vi "NI PXIe-411x PS Main Page.vi"(8 "error in (no error)":errorcluster, 11 "Node Ptr":T1 format="%.0x") -> (0 "error out":errorcluster)   [LabVIEW 2023, in "NI PXIe-411x PS Custom Device.lvlib"]
uses:
  NI PXIe-411x PS Custom Device.lvlib
  <vilib>/NI VeriStand/Custom Device API/Custom Device Item Ref.ctl
  411x_Global.vi
  <vilib>/NI VeriStand/Custom Device API/Get Item Property (String).vi
  <vilib>/NI VeriStand/Custom Device API/Get Item Property (Boolean).vi
  <vilib>/NI VeriStand/Custom Device API/Set Item Property (String).vi
  <vilib>/NI VeriStand/Custom Device API/Set Item Property (Boolean).vi
  <vilib>/NI VeriStand/Custom Device API/Custom Device API.lvlib
panel:
  in  "Module":bool=TRUE
  in  "HW Device Name in MAX":string
  in  "Add Current Chans":bool
  in  "Add Voltage Chans":bool
  in  "Header":cluster{"Section Name":string}={"Section Name"="PXIe-411x  Settings"}
  in  "Description":string
  in  "Custom Device Name":string
  in  "Delete":bool
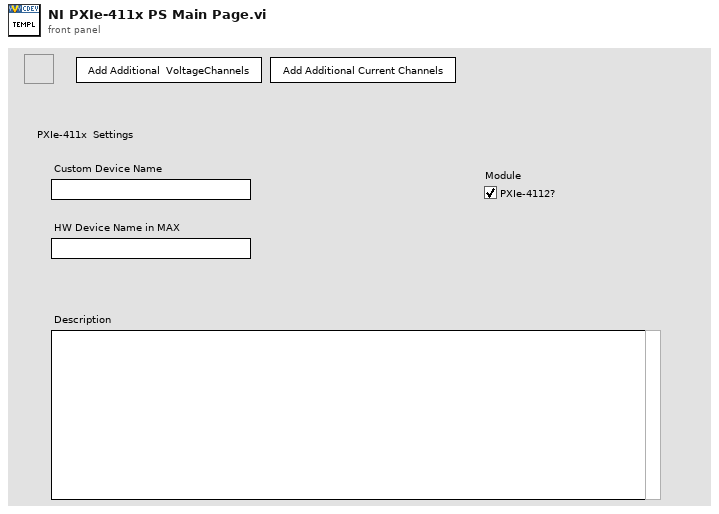
[diagram p1: front panel]
types:
  T1 = typedef "Custom Device API.lvlib/Custom Device Item Ref.ctl" = u64
  T2 = typedef "Custom Device API.lvlib/Custom Device Item Info.ctl" = cluster{"Name":string, "Is Channel":bool, "GUID":string, "Is Waveform":bool}
  T3 = typedef "Custom Device API.lvlib/Custom Device Commands.ctl" = enum16{"Default", "Item renamed", "Shutdown", "Dynamic button pressed"}
  T4 = typedef "niDCPower Sense.ctl" = i32
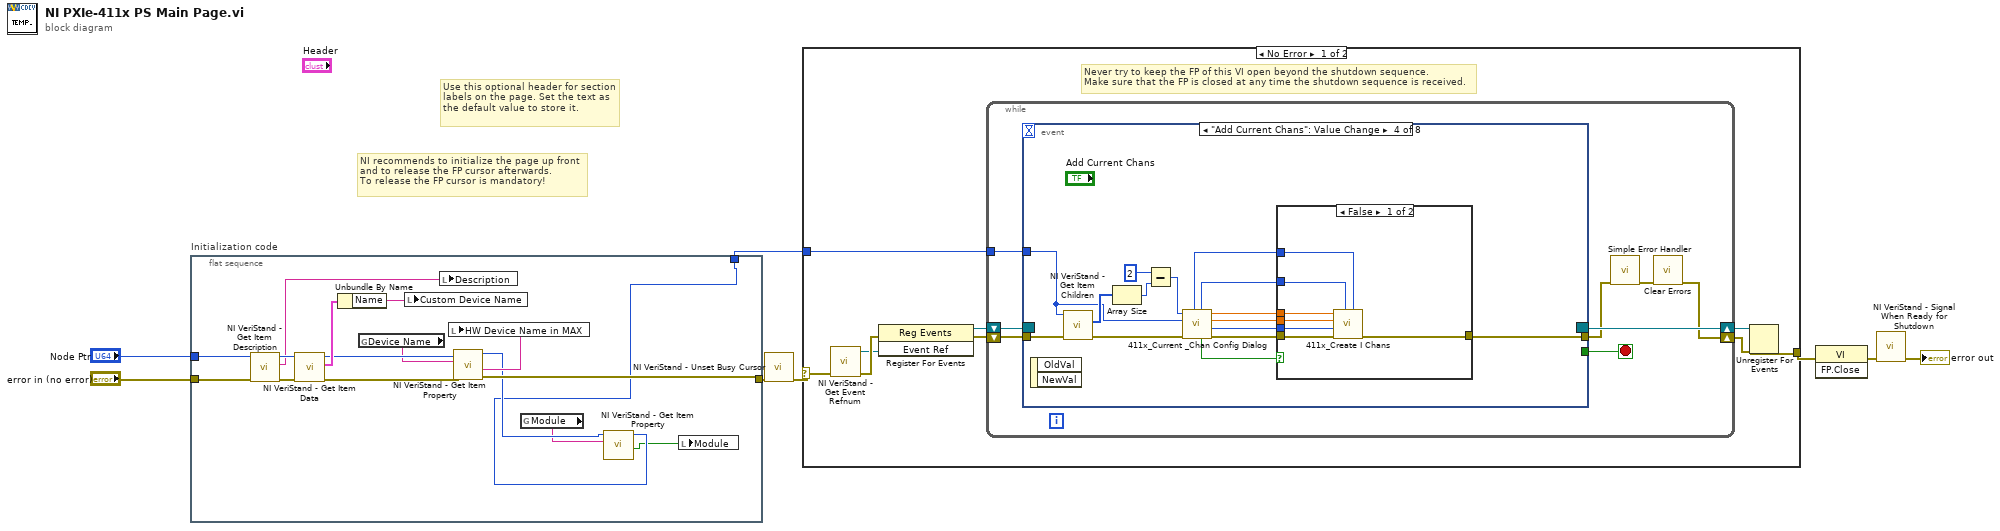
[diagram p0: block diagram]
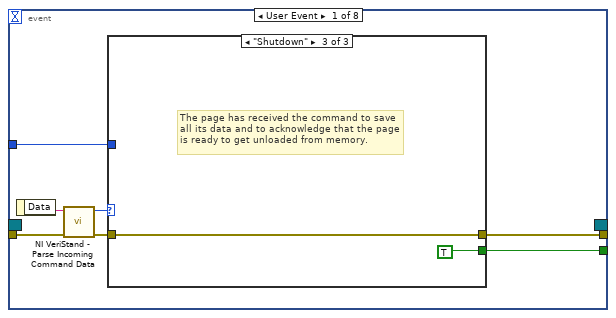
[diagram p2: hidden frame]
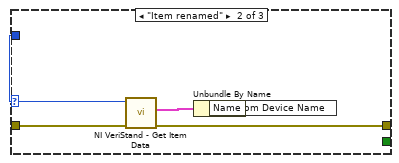
[diagram p4: hidden frame]
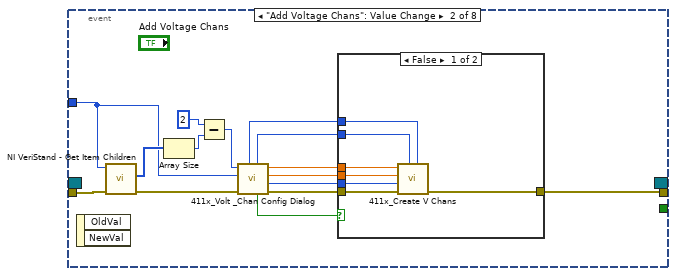
[diagram p5: hidden frame]
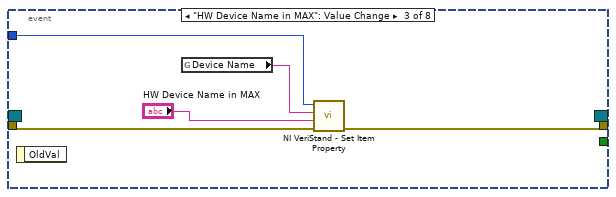
[diagram p7: hidden frame]
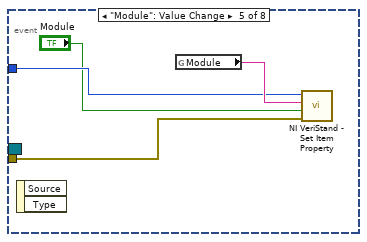
[diagram p9: hidden frame]
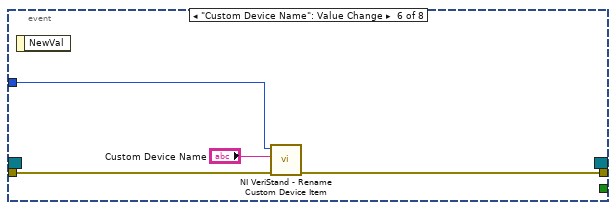
[diagram p10: hidden frame]
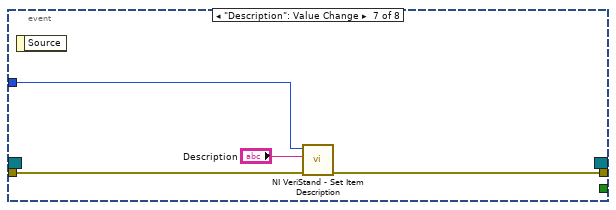
[diagram p11: hidden frame]
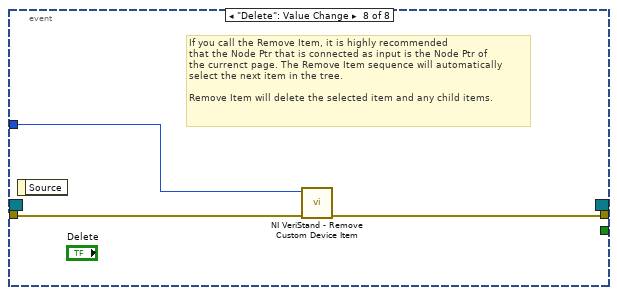
[diagram p12: hidden frame]
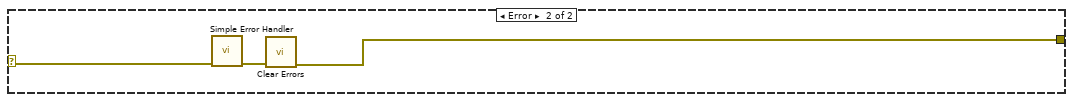
[diagram p13: hidden frame]
diagram:
  # "Use this optional header for section labels on the page. Set the text as the default value to store it."
  # "NI recommends to initialize the page up front\nand to release the FP cursor afterwards.\nTo release the FP cursor is mandatory!"
  n1 = flat-sequence "Initialization code" {
    tunnel: "error in (no error)" -> [w18]
    tunnel: "Node Ptr" -> [w19]
    tunnel: [w15] -> w4
    tunnel: [w11] -> w1
    frame #0 {
      n2 = call <vilib>:"NI VeriStand - Get Item Description.vi"("error in (no error)"=w18, "Item Ref in"=w19) -> ("error out"=w22:errorcluster, "Description"=w23:string, "Item Ref out"=w24:T1)  [unwired: 7 out]
      n3 = call <vilib>:"NI VeriStand - Get Item Data.vi"("error in (no error)"=w22, "Item Ref in"=w24) -> ("error out"=w17:errorcluster, "Item Info"=w21:T2, "Item Ref out"=w16:T1)  [unwired: 7 out]
      n4 = Unbundle By Name(w21) -> ("Name"=w20:string)
      n5 = global read "411x_Global.vi" "Device Name"() -> (w14:string)
      n6 = local write "Custom Device Name"(w20) -> ()
      n7 = local write "Description"(w23) -> ()
      n8 = call-poly <vilib>:"NI VeriStand - Get Item Property.vi"("error in (no error)"=w17, "Property Name"=w14, "Item Ref in"=w16) -> ("error out"=w15:errorcluster, "Value"=w13:string, "Item Ref out"=w12:T1)  [unwired: 5 in, 1 out]
      n9 = local write "HW Device Name in MAX"(w13) -> ()
      n10 = global read "411x_Global.vi" "Module"() -> (w10:string)
      n11 = call-poly <vilib>:"NI VeriStand - Get Item Property.vi"("Property Name"=w10, "Item Ref in"=w12) -> ("Value"=w9:bool, "Item Ref out"=w11:T1)  [unwired: 6 in, 2 out]
      n12 = local write "Module"(w9) -> ()
    }
  }
  n13 = call <vilib>:"NI VeriStand - Unset Busy Cursor.vi"("error in (no error)"=w4) -> ("error out"=w3:errorcluster)  [unwired: 10 out]
  n14 = case shown="No Error" w3 {
    selector: w3 -> [w25 w125]
    tunnel: [w30 w123] -> w8
    tunnel: w1 -> [w26 _]
    frame No Error {
      # "Never try to keep the FP of this VI open beyond the shutdown sequence.\nMake sure that the FP is closed at any time the shutdown sequence is received."
      n15 = call <vilib>:"NI VeriStand - Get Event Refnum.vi"("error in (no error)"=w25) -> ("error out"=w33:errorcluster, "Event Ref"=w29:refnum<user-event>)  [unwired: 9 out]
      n16 = register-events(error in=w33, w29) -> (reference out=w27:refnum<event-registration>, error out=w28:errorcluster)  [unwired: 1 in]
      n17 = while {
        tunnel: w26 -> [w37]
        shift-right: [w34] -> w31
        shift-left: w28 -> [w40]
        shift-right: [w41] -> w32
        shift-left: w27 -> [w39]
        stop <- w38 stop-if-true
        n18 = event shown="[3] \"Add Current Chans\": Value Change" {
          selector: w39 -> [_ _ _ _ _ _ _ _]
          dyn-events: [_ _ _ _ _ _ _ _] -> w41
          timeout: _ -> [_ _ _ _ _ _ _ _]
          tunnel: w40 -> [w48 w71 w84 w99 w108 w115 w118 w122]
          tunnel: [w44 _ _ _ _ _ _ _] -> w38
          tunnel: [w43 w60 w80 w88 _ w114 w117 w121] -> w36
          tunnel: w37 -> [w42 w58 w83 w86 w110 w113 w119 w120]
          event User Event {
            n19 = event-data() -> ("Data"=w47:string)  [unwired: 1 out]
            n20 = call <vilib>:"NI VeriStand - Parse Incoming Command Data.vi"("error in (no error)"=w48, "Incoming data"=w47) -> ("error out"=w46:errorcluster, "Action"=w45:T3)  [unwired: 8 out]
            n21 = case shown="\"Shutdown\"" w45 {
              tunnel: w46 -> [w49 w54 w55]
              tunnel: [_ _ TRUE] -> w44
              tunnel: [w49 w51 w55] -> w43
              tunnel: w42 -> [_ w53 _]
              frame "Default", Default {
              }
              frame "Item renamed" {
                n22 = call <vilib>:"NI VeriStand - Get Item Data.vi"("error in (no error)"=w54, "Item Ref in"=w53) -> ("error out"=w51:errorcluster, "Item Info"=w52:T2)  [unwired: 8 out]
                n23 = Unbundle By Name(w52) -> ("Name"=w50:string)
                n24 = local write "Custom Device Name"(w50) -> ()
              }
              frame "Shutdown" {
                # "The page has received the command to save all its data and to acknowledge that the page is ready to get unloaded from memory."
              }
            }
          }
          event "Add Voltage Chans": Value Change {
            n25 = event-data() -> ()  [unwired: 3 out]
            n26 = call <vilib>:"NI VeriStand - Get Item Children.vi"("error in (no error)"=w71, "Item Ref in"=w58) -> ("error out"=w70:errorcluster, "Child Refs"=w59:T1[])  [unwired: 6 in, 2 out]
            n27 = Array Size(array=w59) -> (size(s)=w68:i32)
            n28 = Subtract(x=2, y=w68) -> (x-y=w67:i32)
            n29 = call "411x_Volt _Chan Config Dialog.vi"("error in (no error)"=w70, "Item Ref out"=w58, "Data Entry Limits:Maximum"=w67) -> ("error out"=w61:errorcluster, "sense (out)"=w62:T4, "Current Limit (out)"=w63:dbl, "Initial Voltage Value (out)"=w64:dbl, "Cancel (out)"=w66:bool, "Number of Voltage Output Channels to Add? (out)"=w65:i16, "Item Ref out"=w57:T1)  [unwired: 2 in]
            n30 = case shown="False" w66 {
              tunnel: w65 -> [w78 _]
              tunnel: w64 -> [w77 _]
              tunnel: w63 -> [w76 _]
              tunnel: w62 -> [w75 _]
              tunnel: w61 -> [w74 w79]
              tunnel: [w73 w79] -> w60
              tunnel: w57 -> [w72 _]
              frame False {
                n31 = call "411x_Create V Chans.vi"("Device Ref in"=w72, "# of V Channels to Add?"=w78, "error in"=w74, "sense"=w75, "Current Limit"=w76, "Init Value"=w77) -> ("error out"=w73:errorcluster)  [unwired: 5 in]
              }
              frame True {
                # "Canceled"
              }
            }
          }
          event "HW Device Name in MAX": Value Change {
            n32 = event-data() -> ()  [unwired: 2 out]
            n33 = global read "411x_Global.vi" "Device Name"() -> (w82:string)
            n34 = call-poly <vilib>:"NI VeriStand - Set Item Property.vi"("error in (no error)"=w84, "Value"="HW Device Name in MAX", "Property Name"=w82, "Item Ref in"=w83) -> ("error out"=w80:errorcluster)  [unwired: 5 in, 2 out]
          }
          event "Add Current Chans": Value Change {
            n35 = event-data() -> ()  [unwired: 3 out]
            n36 = call <vilib>:"NI VeriStand - Get Item Children.vi"("error in (no error)"=w99, "Item Ref in"=w86) -> ("error out"=w98:errorcluster, "Child Refs"=w87:T1[])  [unwired: 6 in, 2 out]
            n37 = Array Size(array=w87) -> (size(s)=w96:i32)
            n38 = Subtract(x=2, y=w96) -> (x-y=w95:i32)
            n39 = call "411x_Current _Chan Config Dialog.vi"("error in (no error)"=w98, "Item Ref out"=w86, "Data Entry Limits:Maximum"=w95) -> ("error out"=w89:errorcluster, "sense (out)"=w90:T4, "Voltage Limit (out)"=w91:dbl, "Initial Current Value (out)"=w92:dbl, "Cancel (out)"=w94:bool, "Number of Current Channels to Add? (out)"=w93:i16, "Item Ref out"=w85:T1)  [unwired: 2 in]
            n40 = case shown="False" w94 {
              tunnel: w85 -> [w106 _]
              tunnel: w93 -> [w105 _]
              tunnel: w92 -> [w104 _]
              tunnel: w91 -> [w103 _]
              tunnel: w90 -> [w102 _]
              tunnel: w89 -> [w101 w107]
              tunnel: [w100 w107] -> w88
              frame False {
                n41 = call "411x_Create I Chans.vi"("Device Ref in"=w106, "# of I Channels to Add?"=w105, "error in"=w101, "sense"=w102, "Voltage Limit"=w103, "Init Value"=w104) -> ("error out"=w100:errorcluster)  [unwired: 5 in]
              }
              frame True {
                # "Canceled"
              }
            }
          }
          event "Module": Value Change {
            n42 = event-data() -> ()  [unwired: 3 out]
            n43 = global read "411x_Global.vi" "Module"() -> (w111:string)
            n44 = call-poly <vilib>:"NI VeriStand - Set Item Property.vi"("error in (no error)"=w108, "Value"="Module", "Property Name"=w111, "Item Ref in"=w110) -> ()  [unwired: 5 in, 3 out]
          }
          event "Custom Device Name": Value Change {
            n45 = event-data() -> ()  [unwired: 2 out]
            n46 = call <vilib>:"NI VeriStand - Rename Custom Device Item.vi"("error in (no error)"=w115, "New Name"="Custom Device Name", "Item Ref in"=w113) -> ("error out"=w114:errorcluster)  [unwired: 1 in, 7 out]
          }
          event "Description": Value Change {
            n47 = event-data() -> ()  [unwired: 2 out]
            n48 = call <vilib>:"NI VeriStand - Set Item Description.vi"("error in (no error)"=w118, "Description"="Description", "Item Ref in"=w119) -> ("error out"=w117:errorcluster)  [unwired: 8 out]
          }
          event "Delete": Value Change {
            # "If you call the Remove Item, it is highly recommended\nthat the Node Ptr that is connected as input is the Node Ptr of\nthe currenct page. The Remove Item sequence will automatically\nselect the next item in the tree.\n\nRemove Item will delete the selected item and any child items."
            n49 = event-data() -> ()  [unwired: 2 out]
            n50 = call <vilib>:"NI VeriStand - Remove Custom Device Item.vi"("error in (no error)"=w122, "Item Ref in"=w120) -> ("error out"=w121:errorcluster)  [unwired: 1 in, 8 out]
          }
        }
        n51 = call <vilib>:"Simple Error Handler.vi"("error in (no error)"=w36) -> ("error out"=w35:errorcluster)  [unwired: 1 in, 7 out]
        n52 = call <vilib>:"Clear Errors.vi"("error in (no error)"=w35) -> ("error out"=w34:errorcluster)  [unwired: 1 in, 5 out]
      }
      n53 = Unregister For Events(event registration refnum=w32, error in=w31) -> (error out=w30:errorcluster)
    }
    frame Error {
      n54 = call <vilib>:"Simple Error Handler.vi"("error in (no error)"=w125) -> ("error out"=w124:errorcluster)  [unwired: 1 in, 7 out]
      n55 = call <vilib>:"Clear Errors.vi"("error in (no error)"=w124) -> ("error out"=w123:errorcluster)  [unwired: 1 in, 5 out]
    }
  }
  n56 = invoke class="VI" method="FP.Close"(error in=w8) -> (error out=w7:errorcluster)  [unwired: 2 in, 2 out]
  n57 = call <vilib>:"NI VeriStand - Signal When Ready for Shutdown.vi"("error in (no error)"=w7) -> ("error out"=→"error out":errorcluster)  [unwired: 10 out]
